vi "Easy Print VI Panel or Documentation (path).vi"(6 "custom contents options":T14 {"list of controls options"."list which controls?" items=["all controls", "connected controls"]}, 7 "layout options":T2={"orientation (unchanged)"=0, "panel scaling for page (unchanged)"=0, "margins"={"override VI margins (false)"=FALSE, "margins (1.00)"={"top"=1.0, "left"=1.0, "right"=1.0, "bottom"=1.0}, "measurement system (default)"=0}, "printer options"={"destination printer name (current)"="", "printing method (unchanged)"=0, "color or monochrome (unchanged)"=0}, "page header options"={"page headers (unchanged)"=0, "page header content options"={"Include VI Name"=TRUE, "Include VI Path"=TRUE, "Include Last Modification Date"=TRUE, "Include Date Printed"=TRUE, "Include Page Number"=TRUE, "Include VI Icon"=TRUE}}} {"page header options"."page headers (unchanged)" items=["Unchanged", "Include page headers", "Do not include page headers"]; "printer options"."color or monochrome (unchanged)" items=["Unchanged", "Color/grayscale", "Monochrome"]; "printer options"."printing method (unchanged)" items=["Unchanged", "Standard", "PostScript", "Bitmap"]; "panel scaling for page (unchanged)" items=["Unchanged", "No Scaling", "Scale front panel to fit"]; "orientation (unchanged)" items=["Unchanged", "portrait", "landscape"]; "margins"."measurement system (default)" items=["Default", "US", "Metric"]; "margins"."margins (1.00)"."right" format="%.2f"; "margins"."margins (1.00)"."bottom" format="%.2f"; "margins"."margins (1.00)"."top" format="%.2f"; "margins"."margins (1.00)"."left" format="%.2f"}, 8 "error in (no error)":errorcluster, 9 "report type (Quick Print)":T1 items=["Quick Print", "Standard Report", "HTML", "Word", "Excel"], 10 "contents (complete front panel)":T16 items=["Complete front panel", "Visible portion of front panel", "Icon, description, panel and diagram", "Documentation: Using the panel", "Documentation: Using as a subVI", "Documentation: Complete", "Documentation: Custom"], 11 "VI path":path) -> (0 "error out":errorcluster, 3 "report out":refnum<class "NI_report.lvclass">)   [LabVIEW 2020, in "NI_ReportGenerationCore.lvlib"]
doc: "This VI is deprecated. Use the following VI instead:\n\nvi.lib\\printing\\EasyPrinting.llb\\Print VI Panel or Documentation.vi\n\nPrints a front panel or VI documentation or saves the front panel or VI documentation to a report. Wire data to the <B>VI path</B> input to determine the polymorphic instance to use or manually select the instance."
uses:
  <vilib>/Utility/NIReport.llb/NI_ReportGenerationCore.lvlib
  <vilib>/printing/EasyPrintingControls.llb/contents.ctl
  <vilib>/printing/EasyPrintingControls.llb/report_type.ctl
  <vilib>/printing/EasyPrintingControls.llb/layout_options.ctl
  <vilib>/printing/EasyPrintingControls.llb/orientation.ctl
  <vilib>/printing/EasyPrintingControls.llb/panel_scaling_for_page.ctl
  <vilib>/printing/EasyPrintingControls.llb/margins.ctl
  <vilib>/printing/EasyPrintingControls.llb/margin_values.ctl
  <vilib>/printing/EasyPrintingControls.llb/measurement_system.ctl
  <vilib>/printing/EasyPrintingControls.llb/printer_options.ctl
  <vilib>/printing/EasyPrintingControls.llb/printing_method.ctl
  <vilib>/printing/EasyPrintingControls.llb/color_or_monochrome.ctl
  <vilib>/printing/EasyPrintingControls.llb/page_header_options.ctl
  <vilib>/printing/EasyPrintingControls.llb/page_headers.ctl
  <vilib>/printing/EasyPrintingControls.llb/page_header_content_options.ctl
  <vilib>/printing/EasyPrintingControls.llb/custom_contents_options.ctl
  <vilib>/printing/EasyPrintingControls.llb/list_which_controls.ctl
  <vilib>/Utility/NIReport.llb/NI_report.lvclass
panel:
  # "This VI is deprecated. Use the following VI instead:\n\nvi.lib\\printing\\EasyPrinting.llb\\Print VI Panel or Documentation.vi"
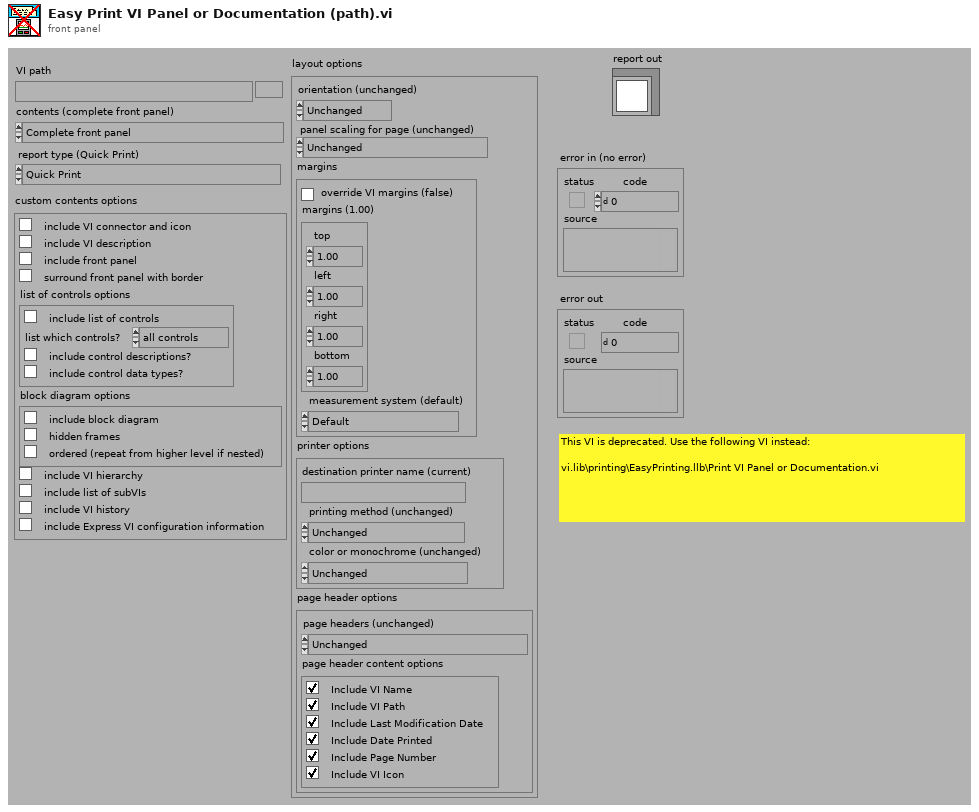
[diagram p1: front panel]
types:
  T1 = typedef "NI_ReportGenerationCore.lvlib/report_type.ctl" = u16
  T2 = typedef "NI_ReportGenerationCore.lvlib/layout_options.ctl" = cluster{"orientation (unchanged)":T3, "panel scaling for page (unchanged)":T4, "margins":T5, "printer options":T8, "page header options":T11}
  T3 = typedef "NI_ReportGenerationCore.lvlib/orientation.ctl" = u16
  T4 = typedef "NI_ReportGenerationCore.lvlib/panel_scaling_for_page.ctl" = u16
  T5 = typedef "NI_ReportGenerationCore.lvlib/margins.ctl" = cluster{"override VI margins (false)":bool, "margins (1.00)":T6, "measurement system (default)":T7}
  T6 = typedef "NI_ReportGenerationCore.lvlib/margin_values.ctl" = cluster{"top":dbl, "left":dbl, "right":dbl, "bottom":dbl}
  T7 = typedef "NI_ReportGenerationCore.lvlib/measurement_system.ctl" = u16
  T8 = typedef "NI_ReportGenerationCore.lvlib/printer_options.ctl" = cluster{"destination printer name (current)":string, "printing method (unchanged)":T9, "color or monochrome (unchanged)":T10}
  T9 = typedef "NI_ReportGenerationCore.lvlib/printing_method.ctl" = u16
  T10 = typedef "NI_ReportGenerationCore.lvlib/color_or_monochrome.ctl" = u16
  T11 = typedef "NI_ReportGenerationCore.lvlib/page_header_options.ctl" = cluster{"page headers (unchanged)":T12, "page header content options":T13}
  T12 = typedef "NI_ReportGenerationCore.lvlib/page_headers.ctl" = u16
  T13 = typedef "NI_ReportGenerationCore.lvlib/page_header_content_options.ctl" = cluster{"Include VI Name":bool, "Include VI Path":bool, "Include Last Modification Date":bool, "Include Date Printed":bool, "Include Page Number":bool, "Include VI Icon":bool}
  T14 = typedef "NI_ReportGenerationCore.lvlib/custom_contents_options.ctl" = cluster{"include VI connector and icon":bool, "include VI description":bool, "include front panel":bool, "surround front panel with border":bool, "list of controls options":cluster{"include list of controls":bool, "list which controls?":T15, "include control descriptions?":bool, "include control data types?":bool}, "block diagram options":cluster{"include block diagram":bool, "hidden frames":bool, "ordered (repeat from higher level if nested)":bool}, "include VI hierarchy":bool, "include list of subVIs":bool, "include VI history":bool, "include Express VI configuration information":bool}
  T15 = typedef "NI_ReportGenerationCore.lvlib/list_which_controls.ctl" = u16
  T16 = typedef "NI_ReportGenerationCore.lvlib/contents.ctl" = u16
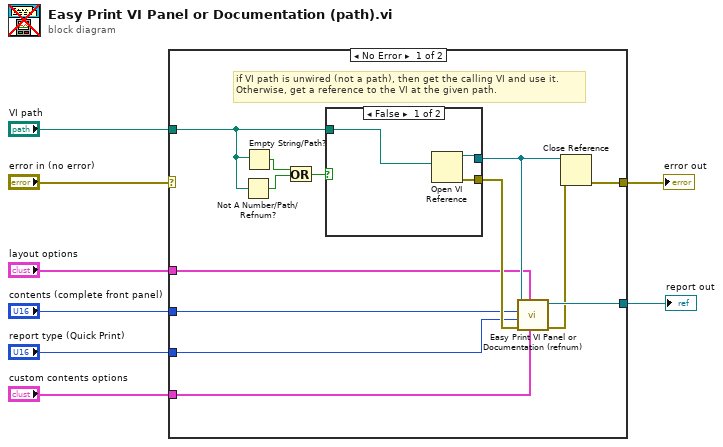
[diagram p0: block diagram]
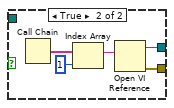
[diagram p2: hidden frame]
diagram:
  n1 = case shown="No Error" "error in (no error)" {
    selector: "error in (no error)" -> [_ w30]
    tunnel: [w16 w30] -> w7
    tunnel: "VI path" -> [w15 _]
    tunnel: "layout options" -> [w14 _]
    tunnel: "contents (complete front panel)" -> [w13 _]
    tunnel: "report type (Quick Print)" -> [w12 _]
    tunnel: "custom contents options" -> [w11 _]
    tunnel: [w10 _] -> w1
    frame No Error {
      # "if VI path is unwired (not a path), then get the calling VI and use it. \nOtherwise, get a reference to the VI at the given path."
      n2 = Not A Number/Path/Refnum?(number/path/refnum=w15) -> (NaN/Path/Refnum?=w20:bool)
      n3 = Empty String/Path?(string/path=w15) -> (empty?=w21:bool)
      n4 = Or(x=w21, y=w20) -> (x .or. y?=w19:bool)
      n5 = case shown="False" w19 {
        tunnel: [w23 w26] -> w17
        tunnel: [w22 w25] -> w18
        tunnel: w15 -> [w24 _]
        frame False {
          n6 = Open VI Reference(vi path=w24) -> (vi reference=w23:refnum<vi>, error out=w22:errorcluster)  [unwired: 5 in]
        }
        frame True {
          n7 = Call Chain() -> (call chain=w29:string[])
          n8 = Index Array(array=w29, index=1 ("Index")) -> (element=w27:string)
          n9 = Open VI Reference(vi path=w27) -> (vi reference=w26:refnum<vi>, error out=w25:errorcluster)  [unwired: 5 in]
        }
      }
      n10 = call <vilib>:"Easy Print VI Panel or Documentation (refnum).vi"("custom contents options"=w11, "layout options"=w14, "error in (no error)"=w18, "report type (Quick Print)"=w12, "contents (complete front panel)"=w13, "VI reference"=w17) -> ("error out"=w9:errorcluster, "report out"=w10:refnum<class "NI_report.lvclass">)  [unwired: 4 in]
      n11 = Close Reference(reference=w17, error in (no error)=w9) -> (error out=w16:errorcluster)
    }
    frame Error {
    }
  }
  "error out" <- w7
  "report out" <- w1
